vi "writeToXML.vi"(8 "error in (no error)":errorcluster, 10 "ClassLabel":string, 11 "TargetOffsetCommands in":refnum<class "TargetOffsetCommands.lvclass">) -> (0 "error out":errorcluster, 2 "XML out":string, 3 "TargetOffsetCommands out":refnum<class "TargetOffsetCommands.lvclass">)   [LabVIEW 2014, in "TCSDataDefinitions.lvlib" / "TCSCommand.lvlib" / "OffsetCommands.lvlib" / "TargetOffsetCommands.lvclass"]
uses:
  TargetOffsetCommands.lvclass
  OffsetCommands/OffsetCommands.lvclass
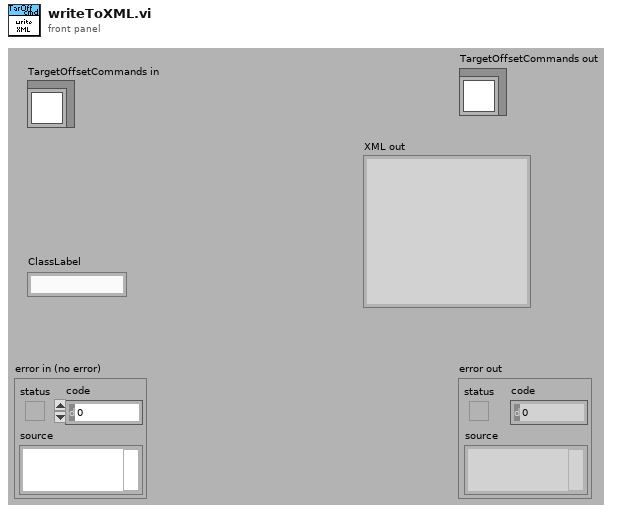
[diagram p1: front panel]
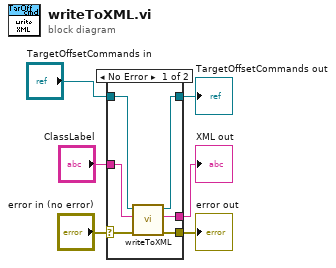
[diagram p0: block diagram]
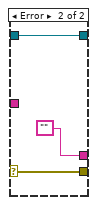
[diagram p2: hidden frame]
diagram:
  n1 = case shown="No Error" "error in (no error)" {
    selector: "error in (no error)" -> [w11 w15]
    tunnel: [w10 w15] -> w5
    tunnel: [w7 w14] -> w4
    tunnel: "TargetOffsetCommands in" -> [w8 w14]
    tunnel: "ClassLabel" -> [w12 _]
    tunnel: [w9 ""] -> w2
    frame No Error {
      n2 = call-parent "writeToXML.vi"("error in (no error)"=w11, "ClassLabel"=w12, "OffsetCommands in"=w8) -> ("error out"=w10:errorcluster, "XML out"=w9:string, "OffsetCommands out"=w7:refnum<class "TargetOffsetCommands.lvclass">)  [unwired: 6 in]
    }
    frame Error {
    }
  }
  "error out" <- w5
  "TargetOffsetCommands out" <- w4
  "XML out" <- w2
